vi "load vi description map.vi"(11 "Path":path=path "D:/github/JKI-State-Machine-Plus/.doc/VI Description.md") -> (0 "text":string, 3 "variant":variant)   [LabVIEW 2014]
uses:
  JKI-State-Machine-Plus.lvlib
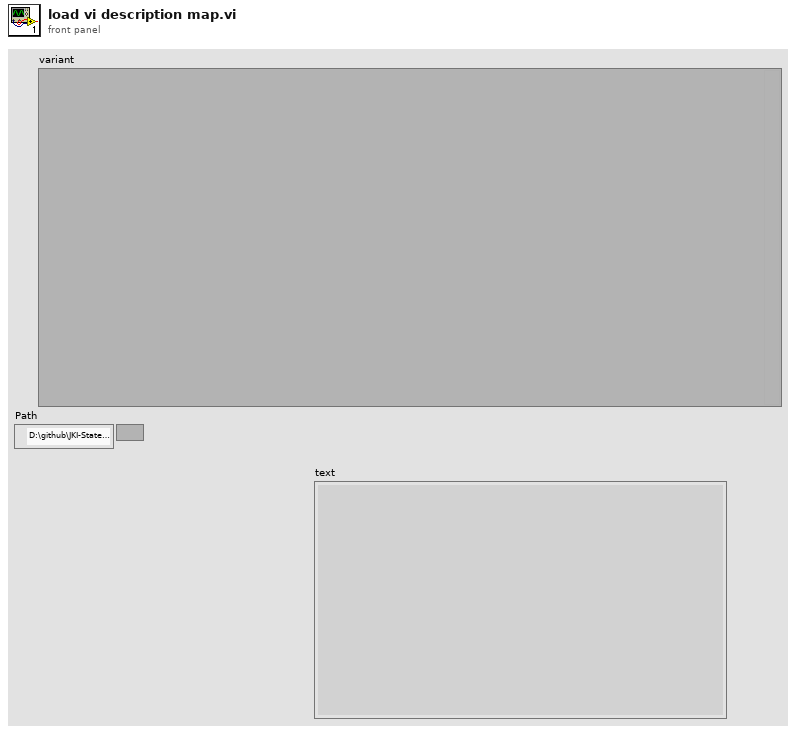
[diagram p1: front panel]
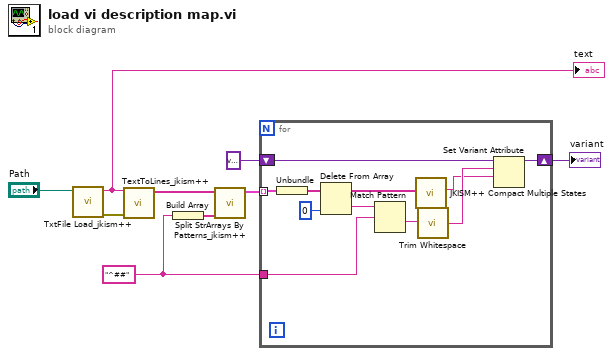
[diagram p0: block diagram]
diagram:
  w4 = "^##" ("delimited string")
  n1 = call "TxtFile Load_jkism++.vi"("Path"="Path") -> ("error out"=w8:errorcluster, "text"=w7:string)  [unwired: 9 in]
  "text" <- w7
  n2 = call "TextToLines_jkism++.vi"("error in (no error)"=w8, "string"=w7) -> ("Lines"=w6:string[])  [unwired: 8 in, 1 out]
  n3 = Build Array(w4) -> (w3:string[])
  n4 = call "Split StrArrays By Patterns_jkism++.vi"("patterns"=w3, "TextArray"=w6) -> ("Array"=w5:cluster{"filtered array":string[]}[])  [unwired: 9 in]
  n5 = for {
    tunnel: w5 -> [w20] mode=indexing
    tunnel: w4 -> [w16]
    shift-right: [w10] -> w1
    shift-left: variant ("variant") -> [w11]
    n6 = Unbundle(w20) -> ("filtered array"=w19:string[])
    n7 = Delete From Array(array=w19, index=0) -> (deleted portion=w17:string, array with subset deleted=w13:string[])  [unwired: 1 in]
    n8 = Match Pattern(string=w17, regular expression=w16) -> (after substring=w15:string)  [unwired: 1 in, 3 out]
    n9 = call "JKISM++ Compact Multiple States.vi"("States in Lines"=w13) -> ("States"=w12:string)  [unwired: 9 in]
    n10 = call <vilib>:"Trim Whitespace.vi"("string"=w15) -> ("trimmed string"=w14:string)  [unwired: 1 in]
    n11 = Set Variant Attribute(Variant=w11, name=w14, value=w12) -> (Variant out=w10:variant)  [unwired: 1 in, 2 out]
  }
  "variant" <- w1
